vi "行列至XY坐标计算.vi"(2 "行位置":i32=1, 3 "列位置":i32=1) -> (0 "纵坐标":dbl, 1 "横坐标":dbl)   [LabVIEW 2020]
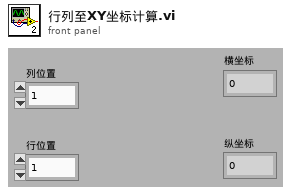
[diagram p1: front panel]
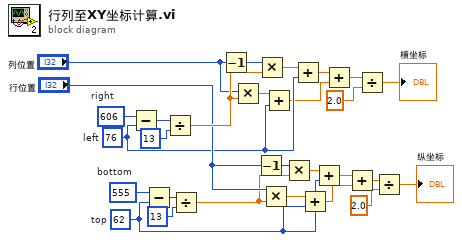
[diagram p0: block diagram]
diagram:
  w25 = i16 555  # bottom
  w12 = i16 62  # top
  w26 = i16 606  # right
  w11 = i16 76  # left
  n1 = Subtract(x=w26, y=w11) -> (x-y=w27:i16)
  n2 = Subtract(x=w25, y=w12) -> (x-y=w23:i16)
  n3 = Divide(x=w27, y=i16 13) -> (x/y=w16:dbl)
  n4 = Divide(x=w23, y=i16 13) -> (x/y=w13:dbl)
  n5 = Decrement(x="列位置") -> (x-1=w22:i32)
  n6 = Multiply(x="列位置", y=w16) -> (x*y=w19:dbl)
  n7 = Decrement(x="行位置") -> (x-1=w21:i32)
  n8 = Multiply(x=w22, y=w16) -> (x*y=w20:dbl)
  n9 = Multiply(x="行位置", y=w13) -> (x*y=w17:dbl)
  n10 = Add(x=w19, y=w11) -> (x+y=w9:dbl)
  n11 = Multiply(x=w21, y=w13) -> (x*y=w18:dbl)
  n12 = Add(x=w20, y=w11) -> (x+y=w10:dbl)
  n13 = Add(x=w17, y=w12) -> (x+y=w7:dbl)
  n14 = Add(x=w18, y=w12) -> (x+y=w8:dbl)
  n15 = Add(x=w10, y=w9) -> (x+y=w6:dbl)
  n16 = Add(x=w8, y=w7) -> (x+y=w5:dbl)
  n17 = Divide(x=w6, y=2.0) -> (x/y=→"横坐标":dbl)
  n18 = Divide(x=w5, y=2.0) -> (x/y=→"纵坐标":dbl)
